vi "SpeedCalc.vi"() -> ()   [LabVIEW 2018]
uses:
  <vilib>/Studica/Studica Toolkit/Background/Mxp Selection.ctl
panel:
  out "x/y":dbl
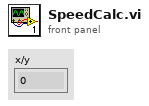
[diagram p1: front panel]
types:
  T1 = typedef "Mxp Selection.ctl" = enum16{"MXP A", "MXP B"}
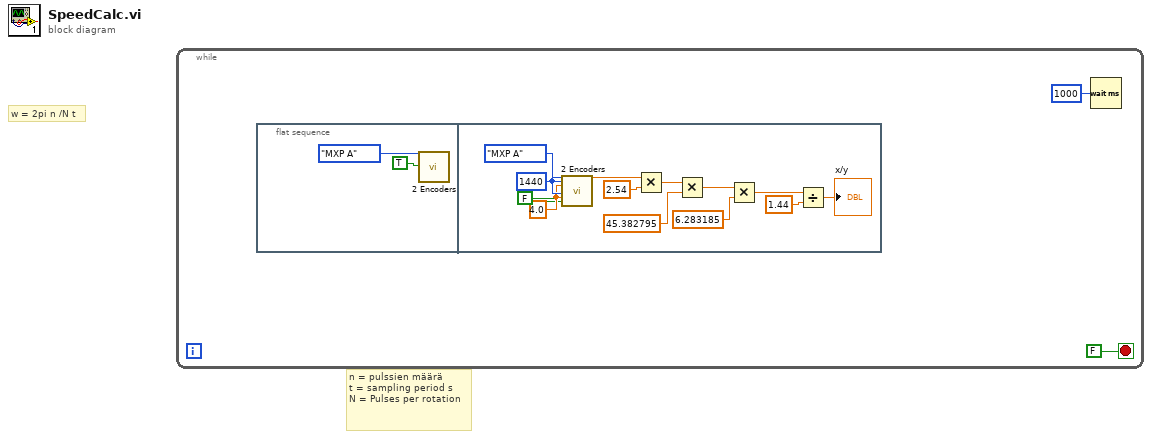
[diagram p0: block diagram]
diagram:
  # "n = pulssien määrä\nt = sampling period s\nN = Pulses per rotation"
  # "w = 2pi n /N t"
  n1 = while {
    stop <- FALSE stop-if-true
    n2 = flat-sequence {
      frame #0 {
        n3 = call <vilib>:"2 Encoders.vi"("Mxp Side"=Mxp_Selection."MXP A", "Reset Encoder 0"=TRUE) -> ()  [unwired: 23 in, 3 out]
      }
      frame #1 {
        w5 = FALSE ("Reset Encoder 0")
        w13 = 4.0 ("Wheel Diameter M1 (inches)")
        w14 = u32 1440 ("Ticks Per Rev M0")
        n4 = call <vilib>:"2 Encoders.vi"("Mxp Side"=Mxp_Selection."MXP A", "Ticks Per Rev M0"=w14, "Wheel Diameter M0 (inches)"=w13, "Reset Encoder 0"=w5, "Ticks Per Rev M1"=w14, "Wheel Diameter M1 (inches)"=w13, "Reset Encoder 1"=w5) -> ("Distance M0 (inches)"=w11:dbl)  [unwired: 18 in, 2 out]
        n5 = Multiply(x=w11, y=2.54) -> (x*y=w16:dbl)
        n6 = Multiply(x=w16, y=45.382795) -> (x*y=w10:dbl)
        n7 = Multiply(x=w10, y=6.283185) -> (x*y=w8:dbl)
        n8 = Divide(x=w8, y=1.44) -> (x/y=→"x/y":dbl)
      }
    }
    n9 = Wait (ms)(milliseconds to wait=u32 1000) -> ()  [unwired: 1 out]
  }
